vi "Begin.vi"(11 "Image Size":T1=enum."160x120") -> (0 "error out":errorcluster)   [LabVIEW 2012]
doc: "Called before other user functions, this VI is expected to open initial I/O refnums, load in file data, and do all program initialization. Notice that the <B>error out</B> terminal is simply used for data flow. Wiring it to other structures or subVIs ensures that this VI runs first."
uses:
  <vilib>/Rock Robotics/WPI/Camera/WPI_CameraImageSize.ctl
  <vilib>/Rock Robotics/WPI/Camera/WPI_CameraWhite Balance Values.ctl
  <vilib>/Rock Robotics/WPI/Camera/WPI_CameraExposure Values.ctl
  <vilib>/Rock Robotics/WPI/Camera/WPI_CameraFrameRate.ctl
  <vilib>/Rock Robotics/WPI/DriverStation/WPI_DriverStationRobotMode2.ctl
  <vilib>/Rock Robotics/SystemInterfaces/DIO/FPGA_DIOChannel.ctl
  <vilib>/Rock Robotics/SystemInterfaces/AI/FPGA_AIGyroChannel.ctl
  <vilib>/Rock Robotics/WPI/Relay/WPI_RelayDirection.ctl
  <vilib>/Rock Robotics/SystemInterfaces/DIO/FPGA_DIORelayChannel.ctl
  <vilib>/Rock Robotics/SystemInterfaces/Typedef/FPGA_TypedefDigitalModule.ctl
  <vilib>/Rock Robotics/SystemInterfaces/AI/FPGA_AIChannel.ctl
  <vilib>/Rock Robotics/SystemInterfaces/DIO/FPGA_DIOPWMChannel.ctl
  <vilib>/Rock Robotics/WPI/Joystick/WPI_JoystickDeviceEnum.ctl
  Robot Global Data.vi
  <vilib>/Rock Robotics/WPI/MotorControl/WPI_MotorControlOpen Victor.vi
  <vilib>/Rock Robotics/WPI/MotorControl/WPI_MotorControlOpen Jaguar.vi
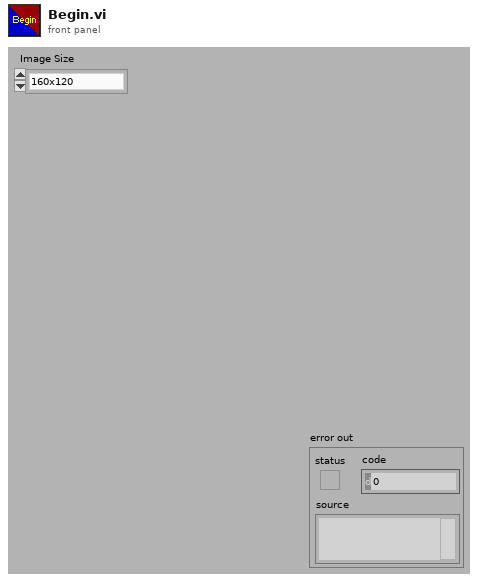
[diagram p1: front panel]
types:
  T1 = typedef "WPI_CameraImageSize.ctl" = enum16{"640x480", "320x240", "160x120"}
  T2 = typedef "WPI_JoystickDeviceEnum.ctl" = enum16{"USB 1", "USB 2", "USB 3", "USB 4", "Kinect 1", "Kinect 2"}
  T3 = typedef "FPGA_TypedefDigitalModule.ctl" = enum16{"Digital Module 1", "Digital Module 2"}
  T4 = typedef "FPGA_DIOPWMChannel.ctl" = enum8{"PWM 1", "PWM 2", "PWM 3", "PWM 4", "PWM 5", "PWM 6", "PWM 7", "PWM 8", "PWM 9", "PWM 10", "Invalid"}
  T5 = typedef "FPGA_AIChannel.ctl" = enum8{"AI 1", "AI 2", "AI 3", "AI 4", "AI 5", "AI 6", "AI 7", "AI 8", "Invalid"}
  T6 = typedef "FPGA_DIOChannel.ctl" = enum8{"DIO 1", "DIO 2", "DIO 3", "DIO 4", "DIO 5", "DIO 6", "DIO 7", "DIO 8", "DIO 9", "DIO 10", "DIO 11", "DIO 12", "DIO 13", "DIO 14", "Invalid"}
  T7 = typedef "FPGA_DIORelayChannel.ctl" = enum8{"Relay 1", "Relay 2", "Relay 3", "Relay 4", "Relay 5", "Relay 6", "Relay 7", "Relay 8", "Invalid"}
  T8 = typedef "WPI_RelayDirection.ctl" = enum16{"Both directions", "Forward only", "Reverse only"}
  T9 = typedef "FPGA_AIGyroChannel.ctl" = enum8{"AI 1", "AI 2", "Invalid"}
  T10 = typedef "WPI_DriverStationRobotMode2.ctl" = enum16{"Autonomous Disabled", "Autonomous Enabled", "Teleop Disabled", "Teleop Enabled", "Timeout", "Finish", "Test Disabled", "Test Enabled"}
  T11 = typedef "WPI_CameraFrameRate.ctl" = u32
  T12 = typedef "WPI_CameraExposure Values.ctl" = enum16{"Auto", "Flicker-free 50 Hz", "Flicker-free 60 Hz", "Hold current"}
  T13 = typedef "WPI_CameraWhite Balance Values.ctl" = enum16{"Auto", "Fixed indoor", "Fixed outdoor 1", "Fixed outdoor 2", "Fixed fluorescent 1", "Fixed fluorescent 2", "Hold current"}
  T14 = typedef "WPI_MotorControlDeviceRef.ctl" = cluster{"DeviceStatus":errorcluster, "Type":enum16{"PWM", "CAN"}, "PWM":cluster{"Digital Module":T3, "PWM Channel":T4, "DeadBand":T15}, "CAN":cluster{"Device Number":u8, "Control Mode":T16, "Semaphore":T17, "Max Vout":dbl}, "Invert":bool, "TransformRef":T18, "InvTransformRef":T18}
  T15 = typedef "WPI_PWMDeadband.ctl" = cluster{"Name":string, "maxPositivePwm":i32, "minPositivePwm":i32, "centerPwm":i32, "maxNegativePwm":i32, "minNegativePwm":i32, "angularRange":u16}
  T16 = typedef "WPI_CANJaguar_ControlMode.ctl" = enum8{"Percent VBus", "Current", "Speed", "Position", "Voltage"}
  T17 = typedef "Semaphore RefNum" = refnum<k1>
  T18 = typedef "WPI_PWMTransform_ConPane.ctl" = refnum<vi>
  T19 = typedef "WPI_ServoDeviceRef.ctl" = cluster{"DeviceStatus":errorcluster, "Digital Module":T3, "PWM Channel":T4, "DeadBand":T15}
  T20 = typedef "WPI_RelayDevRef.ctl" = cluster{"DevStatus":errorcluster, "Relay Channel":T7, "Digital Module":T3, "Relay Direction":T8}
  T21 = typedef "WPI_AnalogChannelDevRef.ctl" = cluster{"DevStatus":errorcluster, "Analog Module":T22, "Analog Channel":T5}
  T22 = typedef "FPGA_TypedefAnalogModule.ctl" = enum16{"Analog Module 1", "Analog Module 2"}
  T23 = typedef "WPI_DigitalInputDevRef.ctl" = cluster{"DevStatus":errorcluster, "DIO Channel":T6, "Digital Module":T3}
  T24 = typedef "WPI_CameraDevRef.ctl" = cluster{"Camera Address":string, "CameraStatus":errorcluster, "Acquire Image Notifier":refnum<notifier>}
  T25 = typedef "WPI_JoystickDevRef.ctl" = cluster{"Device":T2}
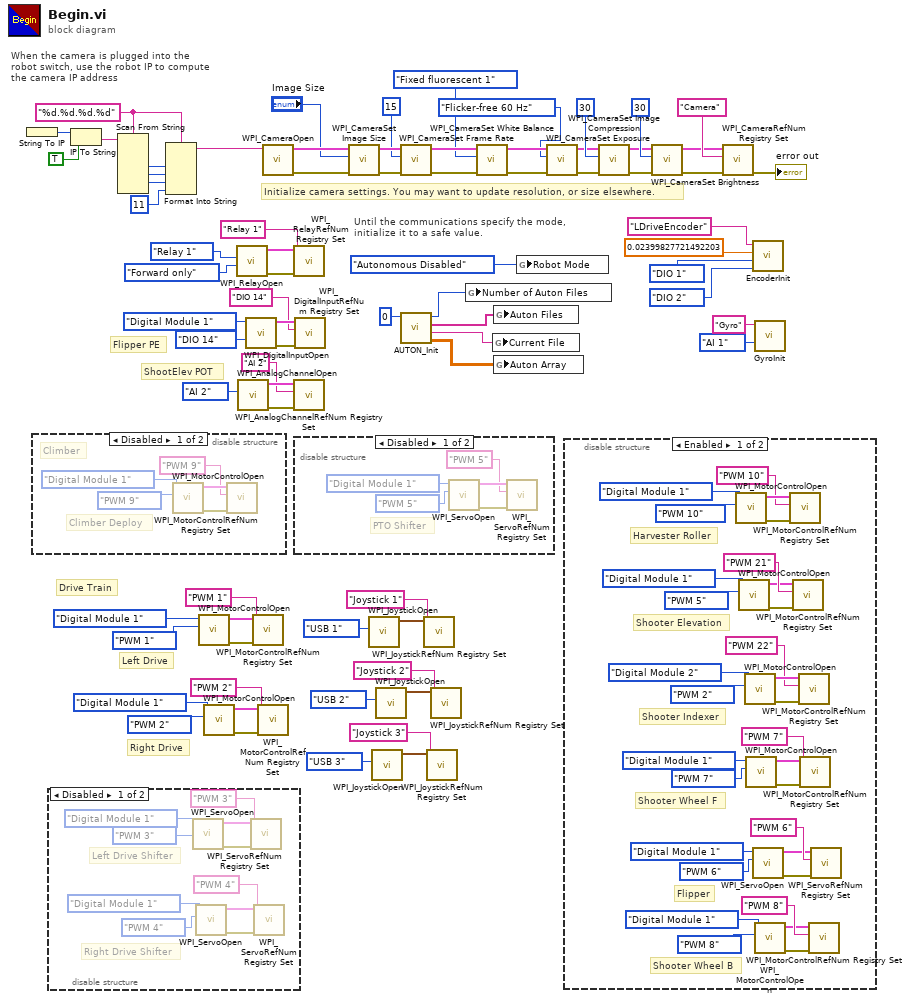
[diagram p0: block diagram]
diagram:
  w48 = "%d.%d.%d.%d" ("format string")
  # "Drive Train"
  # "Right Drive"
  # "Left Drive"
  # "ShootElev POT"
  # "Flipper PE"
  # "Until the communications specify the mode,\ninitialize it to a safe value."
  # "When the camera is plugged into the\nrobot switch, use the robot IP to compute\nthe camera IP address"
  # "Initialize camera settings. You may want to update resolution, or size elsewhere."
  n1 = String To IP() -> (0:w55:u32)  [unwired: 1 in]
  n2 = disable-structure shown="Disabled" {
    frame Disabled {
      # "Climber Deploy"
      # "Climber"
      n3 = call-poly <vilib>:"WPI_MotorControlOpen.vi"("PWM Channel"=FPGA_DIOPWMChannel."PWM 9", "Digital Module (Module 1)"=FPGA_TypedefDigitalModule."Digital Module 1") -> ("error out"=w78:errorcluster, "MotorControlDeviceRef"=w79:T14)  [unwired: 8 in]
      n4 = call <vilib>:"WPI_MotorControlRefNum Registry Set.vi"("error in (no error)"=w78, "refnum name"="PWM 9", "MotorControlDevRef"=w79) -> ()  [unwired: 7 in, 2 out]
    }
    frame Enabled {
    }
  }
  n5 = disable-structure shown="Disabled" {
    frame Disabled {
      # "Right Drive Shifter"
      # "Left Drive Shifter"
      n6 = call <vilib>:"WPI_ServoOpen.vi"("PWM Channel"=FPGA_DIOPWMChannel."PWM 3", "Digital Module (Module 1)"=FPGA_TypedefDigitalModule."Digital Module 1") -> ("error out"=w83:errorcluster, "ServoDeviceRef"=w84:T19)  [unwired: 8 in]
      n7 = call <vilib>:"WPI_ServoOpen.vi"("PWM Channel"=FPGA_DIOPWMChannel."PWM 4", "Digital Module (Module 1)"=FPGA_TypedefDigitalModule."Digital Module 1") -> ("error out"=w82:errorcluster, "ServoDeviceRef"=w89:T19)  [unwired: 8 in]
      n8 = call <vilib>:"WPI_ServoRefNum Registry Set.vi"("error in (no error)"=w83, "refnum name"="PWM 3", "ServoDeviceRef"=w84) -> ()  [unwired: 7 in, 2 out]
      n9 = call <vilib>:"WPI_ServoRefNum Registry Set.vi"("error in (no error)"=w82, "refnum name"="PWM 4", "ServoDeviceRef"=w89) -> ()  [unwired: 7 in, 2 out]
    }
    frame Enabled {
    }
  }
  n10 = IP To String(1:TRUE ("dot notation? (F)"), 2:w55) -> (0:w53:string)
  n11 = Scan From String(format string=w48, input string=w53) -> (output 1=w52:i32, output 2=w51:i32, output 3=w50:i32)  [unwired: 7 in, 3 out]
  n12 = Format Into String(format string=w48, w52, w51, w50, 11 ("Compression")) -> (resulting string=w46:string)  [unwired: 2 in, 1 out]
  n13 = call-poly <vilib>:"WPI_MotorControlOpen.vi"("PWM Channel"=FPGA_DIOPWMChannel."PWM 1", "Digital Module (Module 1)"=FPGA_TypedefDigitalModule."Digital Module 1") -> ("error out"=w10:errorcluster, "MotorControlDeviceRef"=w11:T14)  [unwired: 8 in]
  n14 = call-poly <vilib>:"WPI_MotorControlOpen.vi"("PWM Channel"=FPGA_DIOPWMChannel."PWM 2", "Digital Module (Module 1)"=FPGA_TypedefDigitalModule."Digital Module 1") -> ("error out"=w17:errorcluster, "MotorControlDeviceRef"=w16:T14)  [unwired: 8 in]
  n15 = call <vilib>:"WPI_RelayOpen.vi"("Relay Direction"=WPI_RelayDirection."Forward only", "Relay Channel"=FPGA_DIORelayChannel."Relay 1") -> ("error out"=w33:errorcluster, "RelayDevRef"=w32:T20)  [unwired: 8 in]
  n16 = call <vilib>:"WPI_AnalogChannelOpen.vi"("Analog Channel"=FPGA_AIChannel."AI 2") -> ("error out"=w23:errorcluster, "AIDeviceRef"=w22:T21)  [unwired: 9 in]
  n17 = call <vilib>:"WPI_DigitalInputOpen.vi"("DIO Channel"=FPGA_DIOChannel."DIO 14", "Digital Module (Module 1)"=FPGA_TypedefDigitalModule."Digital Module 1") -> ("error out"=w28:errorcluster, "DigitalInputDevRef"=w27:T23)  [unwired: 8 in]
  n18 = call <vilib>:"WPI_MotorControlRefNum Registry Set.vi"("error in (no error)"=w10, "refnum name"="PWM 1", "MotorControlDevRef"=w11) -> ()  [unwired: 7 in, 2 out]
  n19 = call <vilib>:"WPI_MotorControlRefNum Registry Set.vi"("error in (no error)"=w17, "refnum name"="PWM 2", "MotorControlDevRef"=w16) -> ()  [unwired: 7 in, 2 out]
  n20 = call <vilib>:"WPI_CameraOpen.vi"("Camera Address"=w46) -> ("error out"=w67:errorcluster, "CameraDevRef"=w68:T24)  [unwired: 1 in, 8 out]
  n21 = call <vilib>:"WPI_RelayRefNum Registry Set.vi"("error in (no error)"=w33, "refnum name"="Relay 1", "RelayDevRef"=w32) -> ()  [unwired: 7 in, 2 out]
  n22 = call <vilib>:"WPI_AnalogChannelRefNum Registry Set.vi"("error in (no error)"=w23, "refnum name"="AI 2", "AIDeviceRef"=w22) -> ()  [unwired: 7 in, 2 out]
  n23 = call <vilib>:"WPI_DigitalInputRefNum Registry Set.vi"("error in (no error)"=w28, "refnum name"="DIO 14", "DigitalInputDevRef"=w27) -> ()  [unwired: 7 in, 2 out]
  n24 = disable-structure shown="Disabled" {
    frame Disabled {
      # "PTO Shifter"
      n25 = call <vilib>:"WPI_ServoOpen.vi"("PWM Channel"=FPGA_DIOPWMChannel."PWM 5", "Digital Module (Module 1)"=FPGA_TypedefDigitalModule."Digital Module 1") -> ("error out"=w96:errorcluster, "ServoDeviceRef"=w95:T19)  [unwired: 8 in]
      n26 = call <vilib>:"WPI_ServoRefNum Registry Set.vi"("error in (no error)"=w96, "refnum name"="PWM 5", "ServoDeviceRef"=w95) -> ()  [unwired: 7 in, 2 out]
    }
    frame Enabled {
    }
  }
  n27 = call <vilib>:"WPI_CameraSet Image Size.vi"("error in (no error)"=w67, "Image Size"="Image Size", "CameraDevRef"=w68) -> ("error out"=w66:errorcluster, "CameraDevRef Out"=w69:T24)  [unwired: 7 out]
  n28 = call <vilib>:"WPI_JoystickOpen.vi"("JoystickDevice"=WPI_JoystickDeviceEnum."USB 1") -> ("JoystickDevRef"=w1:T25)  [unwired: 10 in]
  n29 = call <vilib>:"WPI_JoystickOpen.vi"("JoystickDevice"=WPI_JoystickDeviceEnum."USB 3") -> ("JoystickDevRef"=w7:T25)  [unwired: 10 in]
  n30 = call <vilib>:"WPI_JoystickOpen.vi"("JoystickDevice"=WPI_JoystickDeviceEnum."USB 2") -> ("JoystickDevRef"=w6:T25)  [unwired: 10 in]
  n31 = call <vilib>:"WPI_CameraSet Frame Rate.vi"("error in (no error)"=w66, "Frame Rate (fps)"=T11 15, "CameraDevRef"=w69) -> ("error out"=w65:errorcluster, "CameraDevRef Out"=w71:T24)  [unwired: 7 out]
  n32 = call "AUTON_Init.vi"("Default File"=0) -> ("Auton Array"=w40:dbl[][], "Current File"=w41:string, "Auton Files"=w42:string[], "Number of Auton Files"=w43:i64)  [unwired: 7 in]
  n33 = call <vilib>:"WPI_JoystickRefNum Registry Set.vi"("refnum name"="Joystick 1", "JoystickDevRef"=w1) -> ()  [unwired: 8 in, 2 out]
  n34 = call <vilib>:"WPI_JoystickRefNum Registry Set.vi"("refnum name"="Joystick 3", "JoystickDevRef"=w7) -> ()  [unwired: 8 in, 2 out]
  n35 = call <vilib>:"WPI_JoystickRefNum Registry Set.vi"("refnum name"="Joystick 2", "JoystickDevRef"=w6) -> ()  [unwired: 8 in, 2 out]
  n36 = global write "Robot Global Data.vi" "Number of Auton Files"(w43) -> ()
  n37 = call <vilib>:"WPI_CameraSet White Balance.vi"("error in (no error)"=w65, "White Balance"=WPI_CameraWhite_Balance_Values."Fixed fluorescent 1", "CameraDevRef"=w71) -> ("error out"=w64:errorcluster, "CameraDevRef Out"=w70:T24)  [unwired: 7 out]
  n38 = global write "Robot Global Data.vi" "Current File"(w41) -> ()
  n39 = global write "Robot Global Data.vi" "Auton Files"(w42) -> ()
  n40 = global write "Robot Global Data.vi" "Auton Array"(w40) -> ()
  n41 = global write "Robot Global Data.vi" "Robot Mode"(WPI_DriverStationRobotMode2."Autonomous Disabled" ("Robot Mode")) -> ()
  n42 = call <vilib>:"WPI_CameraSet Exposure.vi"("error in (no error)"=w64, "Exposure"=WPI_CameraExposure_Values."Flicker-free 60 Hz", "CameraDevRef"=w70) -> ("error out"=w63:errorcluster, "CameraDevRef Out"=w73:T24)  [unwired: 7 out]
  n43 = disable-structure shown="Enabled" {
    frame Enabled {
      # "Shooter Wheel B"
      # "Flipper"
      # "Shooter Indexer"
      # "Shooter Elevation"
      # "Harvester Roller"
      # "Shooter Wheel F"
      n44 = call-poly <vilib>:"WPI_MotorControlOpen.vi"("PWM Channel"=FPGA_DIOPWMChannel."PWM 10", "Digital Module (Module 1)"=FPGA_TypedefDigitalModule."Digital Module 1") -> ("error out"=w120:errorcluster, "MotorControlDeviceRef"=w121:T14)  [unwired: 8 in]
      n45 = call-poly <vilib>:"WPI_MotorControlOpen.vi"("PWM Channel"=FPGA_DIOPWMChannel."PWM 5", "Digital Module (Module 1)"=FPGA_TypedefDigitalModule."Digital Module 1") -> ("error out"=w114:errorcluster, "MotorControlDeviceRef"=w113:T14)  [unwired: 8 in]
      n46 = call-poly <vilib>:"WPI_MotorControlOpen.vi"("PWM Channel"=FPGA_DIOPWMChannel."PWM 2", "Digital Module (Module 1)"=FPGA_TypedefDigitalModule."Digital Module 2") -> ("error out"=w109:errorcluster, "MotorControlDeviceRef"=w110:T14)  [unwired: 8 in]
      n47 = call-poly <vilib>:"WPI_MotorControlOpen.vi"("PWM Channel"=FPGA_DIOPWMChannel."PWM 7", "Digital Module (Module 1)"=FPGA_TypedefDigitalModule."Digital Module 1") -> ("error out"=w123:errorcluster, "MotorControlDeviceRef"=w124:T14)  [unwired: 8 in]
      n48 = call <vilib>:"WPI_ServoOpen.vi"("PWM Channel"=FPGA_DIOPWMChannel."PWM 6", "Digital Module (Module 1)"=FPGA_TypedefDigitalModule."Digital Module 1") -> ("error out"=w102:errorcluster, "ServoDeviceRef"=w103:T19)  [unwired: 8 in]
      n49 = call-poly <vilib>:"WPI_MotorControlOpen.vi"("PWM Channel"=FPGA_DIOPWMChannel."PWM 8", "Digital Module (Module 1)"=FPGA_TypedefDigitalModule."Digital Module 1") -> ("error out"=w99:errorcluster, "MotorControlDeviceRef"=w98:T14)  [unwired: 8 in]
      n50 = call <vilib>:"WPI_MotorControlRefNum Registry Set.vi"("error in (no error)"=w120, "refnum name"="PWM 10", "MotorControlDevRef"=w121) -> ()  [unwired: 7 in, 2 out]
      n51 = call <vilib>:"WPI_MotorControlRefNum Registry Set.vi"("error in (no error)"=w114, "refnum name"="PWM 21", "MotorControlDevRef"=w113) -> ()  [unwired: 7 in, 2 out]
      n52 = call <vilib>:"WPI_MotorControlRefNum Registry Set.vi"("error in (no error)"=w109, "refnum name"="PWM 22", "MotorControlDevRef"=w110) -> ()  [unwired: 7 in, 2 out]
      n53 = call <vilib>:"WPI_MotorControlRefNum Registry Set.vi"("error in (no error)"=w123, "refnum name"="PWM 7", "MotorControlDevRef"=w124) -> ()  [unwired: 7 in, 2 out]
      n54 = call <vilib>:"WPI_MotorControlRefNum Registry Set.vi"("error in (no error)"=w99, "refnum name"="PWM 8", "MotorControlDevRef"=w98) -> ()  [unwired: 7 in, 2 out]
      n55 = call <vilib>:"WPI_ServoRefNum Registry Set.vi"("error in (no error)"=w102, "refnum name"="PWM 6", "ServoDeviceRef"=w103) -> ()  [unwired: 7 in, 2 out]
    }
    frame Disabled {
    }
  }
  n56 = call <vilib>:"WPI_CameraSet Image Compression.vi"("error in (no error)"=w63, "Compression"=30, "CameraDevRef"=w73) -> ("error out"=w62:errorcluster, "CameraDevRef Out"=w72:T24)  [unwired: 7 out]
  n57 = call <vilib>:"WPI_CameraSet Brightness.vi"("error in (no error)"=w62, "Brightness"=30, "CameraDevRef"=w72) -> ("error out"=w60:errorcluster, "CameraDevRef Out"=w61:T24)  [unwired: 7 out]
  n58 = call <vilib>:"WPI_CameraRefNum Registry Set.vi"("error in (no error)"=w60, "refnum name"="Camera", "CameraDevRef"=w61) -> ("error out"=→"error out":errorcluster)  [unwired: 8 out]
  n59 = call "EncoderInit.vi"("refnum name"="LDriveEncoder", "DistancePerCount"=0.02399827721492203, "DIO Channel"=FPGA_DIOChannel."DIO 1", "DIO Channel 2"=FPGA_DIOChannel."DIO 2") -> ()  [unwired: 7 in]
  n60 = call "GyroInit.vi"("refnum name"="Gyro", "Analog Channel"=FPGA_AIGyroChannel."AI 1") -> ()  [unwired: 8 in]
